vi "tmp.vi"(11 "XYGraph Refnum":refnum<vi>) -> (2 "resulting string":string)   [LabVIEW 2014, in "Graph.lvclass"]
uses:
  Graph.lvclass
  <vilib>/Analysis/1siggen.llb/Ramp Pattern by Samples.vi
  <userlib>/_OpenG.lib/array/array.llb/Remove Duplicates from 1D Array (U32)__ogtk.vi
  <userlib>/_OpenG.lib/array/array.llb/Delete Elements from 1D Array (String)__ogtk.vi
  <vilib>/gmath/NI_Gmath.lvlib
  <vilib>/Analysis/NI_AALBase.lvlib
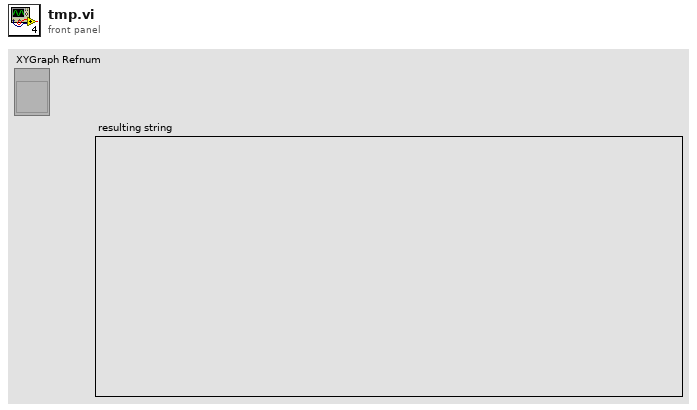
[diagram p1: front panel]
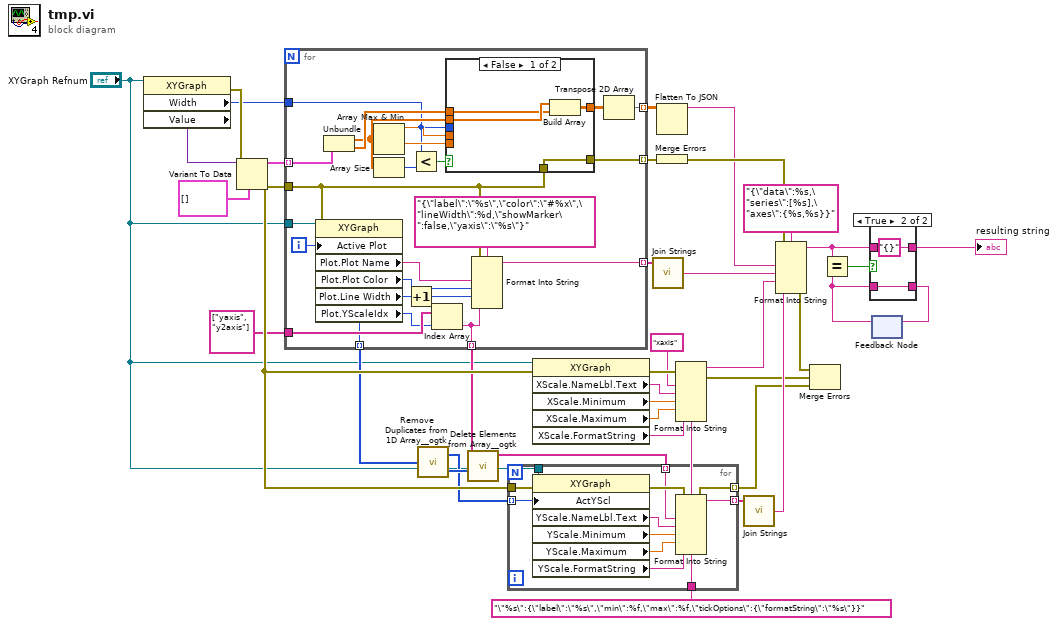
[diagram p0: block diagram]
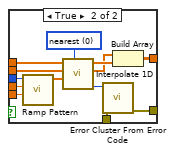
[diagram p3: hidden frame]
diagram:
  w10 = "\"%s\":{\"label\":\"%s\",\"min\":%f,\"max\":%f,\"tickOptions\":{\"formatString\":\"%s\"}}"
  n1 = property class="XYGraph"(reference="XYGraph Refnum") -> (error out=w38:errorcluster, "Width"=w9:u32, "Value"=w34:variant)  [unwired: 1 in, 1 out]
  n2 = Variant To Data(error in=w38, type=cluster{dbl[], dbl[]}[] [], Variant=w34) -> (data=w32:cluster{dbl[], dbl[]}[], error out=w37:errorcluster)
  n3 = for {
    tunnel: [w59] -> w12 mode=indexing
    tunnel: w32 -> [w56] mode=indexing
    tunnel: "XYGraph Refnum" -> [w43]
    tunnel: [w61] -> w31 mode=indexing
    tunnel: w9 -> [w50]
    tunnel: w37 -> [w60]
    tunnel: string[] ["yaxis", "y2axis"] -> [w44]
    tunnel: [w42] -> w16 mode=indexing
    tunnel: [w41] -> w15 mode=indexing
    tunnel: [w40] -> w14 mode=indexing
    i -> [w45]
    n4 = property on="Property Node" class="XYGraph"(reference=w43, error in=w60, "Active Plot"=w45) -> ("Plot.Plot Name"=w47:string, "Plot.Plot Color"=w48:u32, "Plot.Line Width"=w49:u8, "Plot.YScaleIdx"=w42:u32)  [unwired: 2 out]
    n5 = Unbundle(w56) -> (w52:dbl[], w57:dbl[])
    n6 = Array Max & Min(array=w52) -> (max value=w55:dbl, min value=w54:dbl)  [unwired: 2 out]
    n7 = Array Size(array=w52) -> (size(s)=w51:i32)
    n8 = Increment(x=w49) -> (x+1=w39:u8)
    n9 = Less?(x=w50, y=w51) -> (x < y?=w53:bool)
    n10 = Index Array(array=w44, index=w42) -> (element=w41:string)
    n11 = case shown="False" w53 {
      tunnel: [w62 w78] -> w61
      tunnel: [w65 w76] -> w58
      tunnel: w57 -> [w63 w75]
      tunnel: w52 -> [w64 w69]
      tunnel: w55 -> [_ w68]
      tunnel: w54 -> [_ w67]
      tunnel: w50 -> [_ w66]
      tunnel: w60 -> [w62 w77]
      frame False {
        n12 = Build Array(w64, w63) -> (w65:dbl[][])
      }
      frame True {
        w70 = 0 items=["nearest", "linear", "spline", "cubic Hermite", "Lagrange"] ("method")
        n13 = call-poly <vilib>:"Ramp Pattern.vi"("start"=w67, "end"=w68, "samples"=w66) -> ("Ramp Pattern"=w71:dbl[])  [unwired: 7 in, 1 out]
        n14 = call <vilib>:"Interpolate 1D.vi"("method"=w70, "xi"=w71, "X"=w69, "Y"=w75) -> ("error"=w72:i32, "xi used"=w73:dbl[], "yi"=w74:dbl[])  [unwired: 5 in]
        n15 = call <vilib>:"Error Cluster From Error Code.vi"("error in (no error)"=w77, "error code (0)"=w72) -> ("error out"=w78:errorcluster)  [unwired: 7 in]
        n16 = Build Array(w73, w74) -> (w76:dbl[][])
      }
    }
    n17 = Format Into String(format string="{\"label\":\"%s\",\"color\":\"#%x\",\"lineWidth\":%d,\"showMarker\":false,\"yaxis\":\"%s\"}", error in=w60, w47, w48, w39, w41) -> (resulting string=w40:string)  [unwired: 1 in, 1 out]
    n18 = Transpose 2D Array(2D array=w58) -> (transposed array=w59:dbl[][])
  }
  n19 = call-poly <userlib>:"Remove Duplicates from 1D Array__ogtk.vi"("Input Array"=w16) -> ("Output Array"=w17:u32[], "indices of removed elements"=w28:i32[])
  n20 = call-poly <userlib>:"Delete Elements from Array__ogtk.vi"("indices"=w28, "array"=w15) -> ("array w/ subset deleted"=w29:string[])  [unwired: 8 in, 1 out]
  n21 = for {
    tunnel: w17 -> [w88] mode=indexing
    tunnel: w29 -> [w86] mode=indexing
    tunnel: [w82] -> w18 mode=indexing
    tunnel: w10 -> [w81]
    tunnel: "XYGraph Refnum" -> [w80]
    tunnel: w37 -> [w90]
    tunnel: [w79] -> w3 mode=indexing
    n22 = property on="Property Node" class="XYGraph"(reference=w80, error in=w90, "ActYScl"=w88) -> (error out=w89:errorcluster, "YScale.NameLbl.Text"=w87:string, "YScale.Minimum"=w85:dbl, "YScale.Maximum"=w84:dbl, "YScale.FormatString"=w83:string)  [unwired: 1 out]
    n23 = Format Into String(format string=w81, error in=w89, w86, w87, w85, w84, w83) -> (resulting string=w82:string, error out=w79:errorcluster)  [unwired: 1 in]
  }
  n24 = property on="Property Node" class="XYGraph"(reference="XYGraph Refnum", error in=w37) -> (error out=w36:errorcluster, "XScale.NameLbl.Text"=w22:string, "XScale.Minimum"=w23:dbl, "XScale.Maximum"=w24:dbl, "XScale.FormatString"=w25:string)  [unwired: 1 out]
  n25 = call <vilib>:"Join Strings.vi"("Strings In"=w14) -> ("String"=w21:string)  [unwired: 2 in]
  n26 = Flatten To JSON(anything=w12) -> (JSON string=w11:string)  [unwired: 2 in, 1 out]
  n27 = Merge Errors(w31) -> (w35:errorcluster)
  n28 = Format Into String(format string=w10, error in=w36, "xaxis", w22, w23, w24, w25) -> (resulting string=w26:string, error out=w2:errorcluster)  [unwired: 1 in]
  n29 = call <vilib>:"Join Strings.vi"("Strings In"=w18) -> ("String"=w20:string)  [unwired: 2 in]
  n30 = Format Into String(format string="{\"data\":%s,\"series\":[%s],\"axes\":{%s,%s}}", error in=w35, w11, w21, w26, w20) -> (resulting string=w5:string, error out=w1:errorcluster)  [unwired: 1 in]
  n31 = Merge Errors(w1, w2, w3) -> ()  [unwired: 1 out]
  n32 = feedback #1() -> (w6:string)  [unwired: 1 in]
  n33 = Equal?(x=w5, y=w6) -> (x = y?=w8:bool)
  n34 = case shown="True" w8 {
    tunnel: [w91 w93] -> w7
    tunnel: w6 -> [_ w93]
    tunnel: w5 -> [w91 _]
    tunnel: [w91 "{}"] -> w4
    frame False {
    }
    frame True {
    }
  }
  "resulting string" <- w4
  n35 = feedback-in #1(w7) -> ()
